vi "Measurement Logic.vi"(8 "error in":errorcluster, 9 "measurement configuration":T2 {"PAYLOAD" format="%x"; "TYPE" items=["CAN Data"=0, "CAN Remote"=1, "CAN Bus Error"=2, "CAN 2.0 Data"=8, "CAN FD Data"=16, "CAN FD+BRS Data"=24, "J1939 Data"=192, "Delay"=224, "Log Trigger"=225, "Start Trigger"=226]; "IDENTIFIER" format="%x"; "Baudrate" format="%x"; "FD Baudrate" format="%x"}, 10 "measure call context in":refnum<class "Measure Call Context.lvclass">) -> (0 "error out":errorcluster, 1 "measurement results":T1, 2 "measure call context out":refnum<class "Measure Call Context.lvclass">)   [LabVIEW 2025, in "CAN-LIN Frame Generator.lvclass"]
doc: "Contains the core logic for executing the measurement."
uses:
  CAN-LIN Frame Generator.lvclass
  <vilib>/Plug-In SDKs/Measurements/Measure Call Context/Measure Call Context.lvclass
  Measurement Configuration.ctl
  Measurement Results.ctl
  <vilib>/xnet/xnet.llb/XNET Frame CAN.ctl
  <vilib>/xnet/xnet.llb/XNET Frame Type CAN.ctl
  <vilib>/xnet/xnet.llb/XNET Create Session (Frame Output Stream).vi
  <vilib>/xnet/xnet.llb/XNET Write (Frame CAN).vi
  <vilib>/xnet/xnet.llb/XNET Wait (Transmit Complete).vi
  <extravilib>/ChannelInstances/Event Messenger-bool/Instantiate.vi
  <resource>/objmgr/xnet.rc
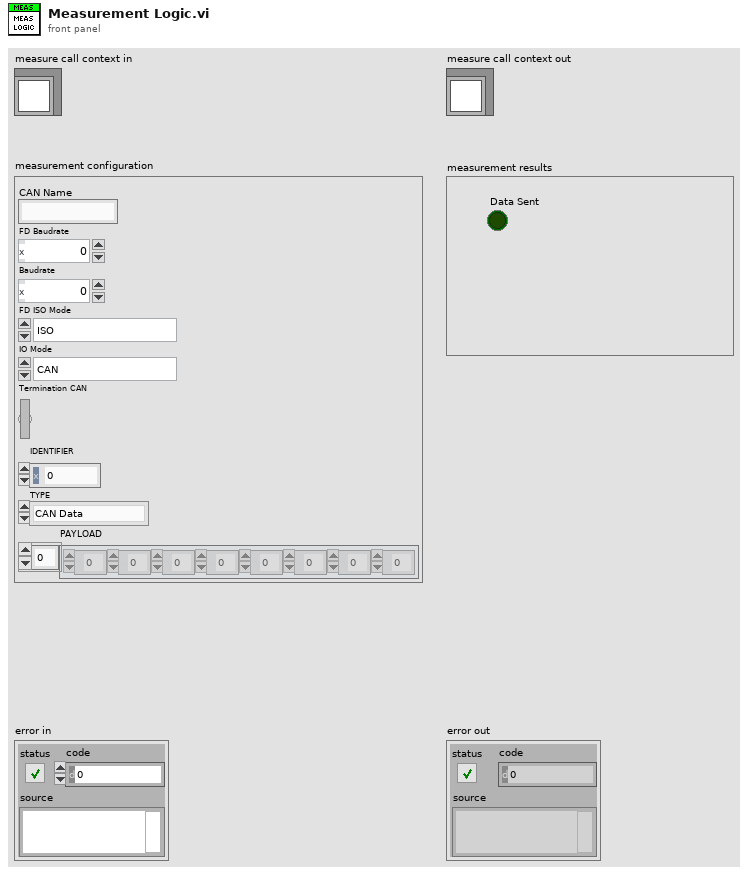
[diagram p1: front panel]
types:
  T1 = typedef "CAN-LIN Frame Generator.lvclass/Measurement Results.ctl" = cluster{"Data Sent":bool}
  T2 = typedef "CAN-LIN Frame Generator.lvclass/Measurement Configuration.ctl" = cluster{"CAN Name ":string, "FD Baudrate":u32, "Baudrate":u32, "FD ISO Mode":enum32{"ISO", "Legacy ISO", "Non-ISO"}, "IO Mode":enum32{"CAN", "CAN FD", "CAN FD + BRS"}, "Termination CAN":bool, "IDENTIFIER":u32, "TYPE":u32, "PAYLOAD":u32[]}
  T3 = typedef "XNET Frame CAN.ctl" = cluster{"timestamp":timestamp, "payload":u8[], "identifier":u32, "type":T4, "extended?":bool, "echo?":bool}
  T4 = typedef "XNET Frame Type CAN.ctl" = u8
  T5 = typedef "Event Messenger-bool.lvlib/))Channel.ctl" = refnum<queue>
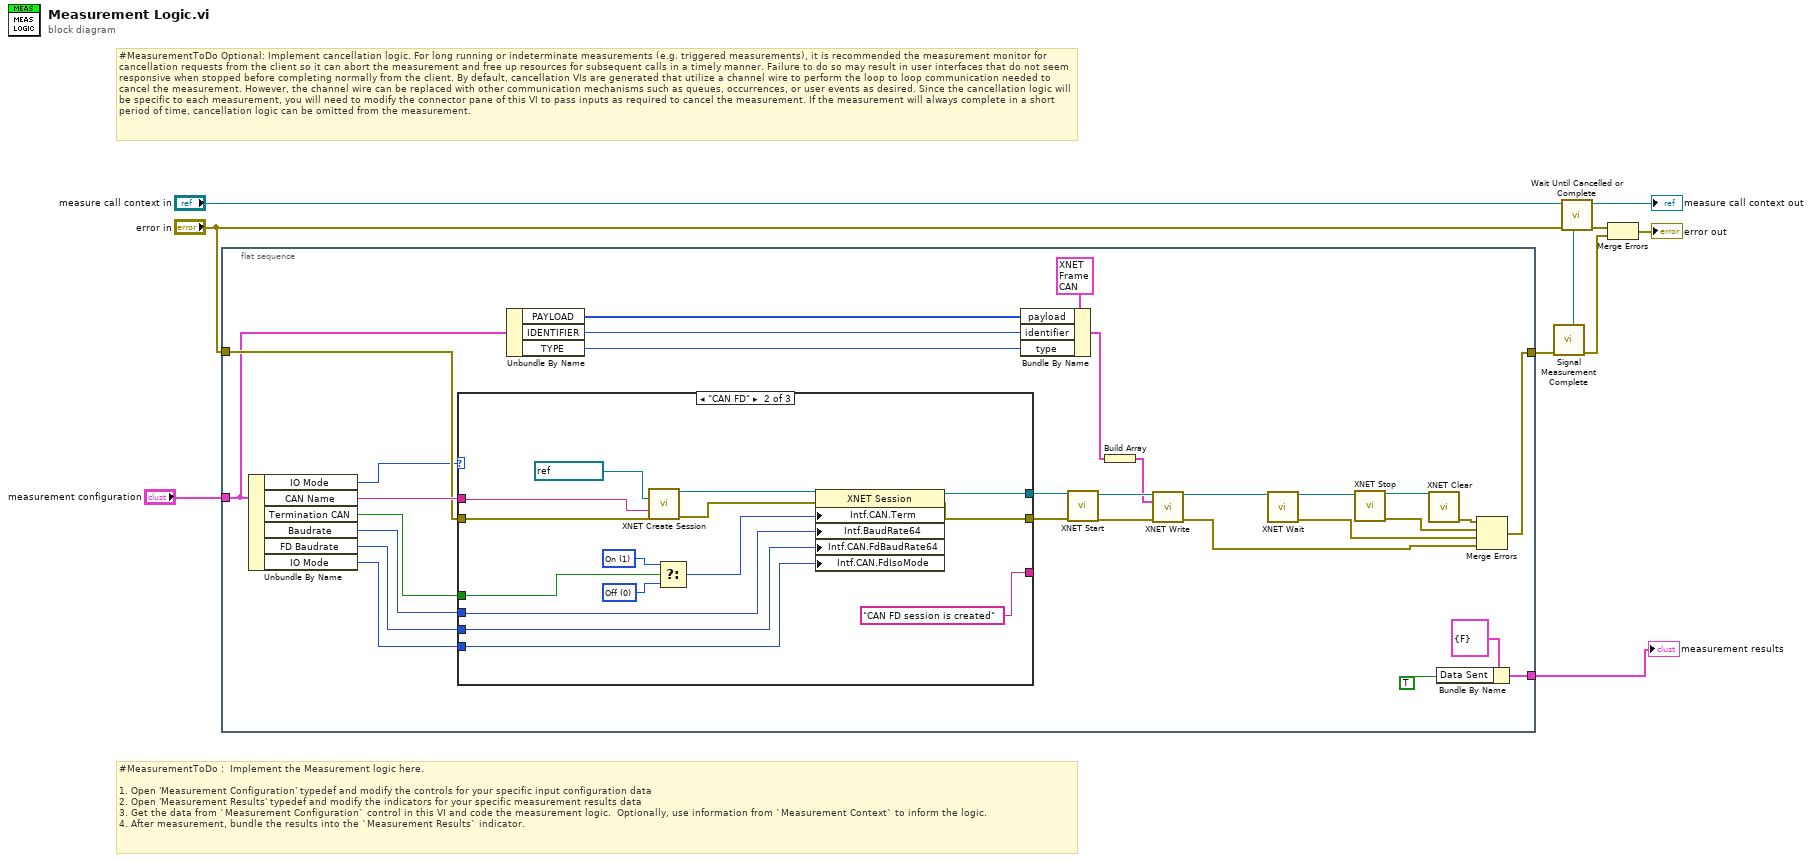
[diagram p0: block diagram]
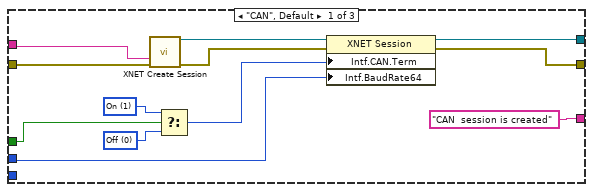
[diagram p2: hidden frame]
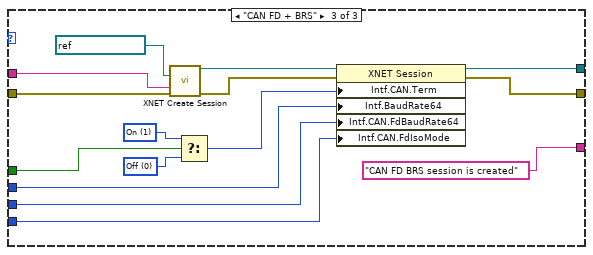
[diagram p3: hidden frame]
diagram:
  # "#MeasurementToDo Optional: Implement cancellation logic. For long running or indeterminate measurements (e.g. triggered measurements), it is recommended the measurement monitor for cancellation requests from the client so it can abort the measurement and free up resources for subsequent calls in a timely manner. Failure to do so may result in user interfaces that do not seem responsive when stopped before completing normally from the client. By default, cancellation VIs are generated that utilize a channel wire to perform the loop to loop communication needed to cancel the measurement. However, the channel wire can be replaced with other communication mechanisms such as queues, occurrences, or user events as desired. Since the cancellation logic will be specific to each measurement, you will need to modify the connector pane of this VI to pass inputs as required to cancel the measurement. If the measurement will always complete in a short period of time, cancellation logic can be omitted from the measurement."
  # "#MeasurementToDo :  Implement the Measurement logic here.\n\n1. Open 'Measurement Configuration' typedef and modify the controls for your specific input configuration data\n2. Open 'Measurement Results' typedef and modify the indicators for your specific measurement results data\n3. Get the data from `Measurement Configuration` control in this VI and code the measurement logic.  Optionally, use information from `Measurement Context` to inform the logic.\n4. After measurement, bundle the results into the `Measurement Results` indicator."
  n1 = flat-sequence {
    tunnel: "measurement configuration" -> [w14]
    tunnel: "error in" -> [w38]
    tunnel: [w16] -> w6
    tunnel: [w28] -> w1
    frame #0 {
      n2 = Unbundle By Name(w14) -> ("IO Mode"=w26:enum32{"CAN", "CAN FD", "CAN FD + BRS"}, "CAN Name"=w39:string, "Termination CAN"=w37:bool, "Baudrate"=w36:u32, "FD Baudrate"=w35:u32, "IO Mode"=w34:enum32{"CAN", "CAN FD", "CAN FD + BRS"})
      n3 = case shown="\"CAN FD\"" w26 {
        tunnel: [w46 w55 w75] -> w33
        tunnel: w39 -> [w41 w60 w70]
        tunnel: w38 -> [w45 w59 w69]
        tunnel: [w44 w54 w68] -> w32
        tunnel: w37 -> [w43 w58 w74]
        tunnel: w36 -> [w42 w57 w73]
        tunnel: w35 -> [_ w53 w72]
        tunnel: w34 -> [_ w56 w71]
        tunnel: ["CAN  session is created" ("message") "CAN FD session is created" ("message") "CAN FD BRS session is created" ("message")] -> _
        frame "CAN", Default {
          w49 = u32 1 items=["Off", "On"] ("Interface:CAN:Termination")
          w48 = u32 0 items=["Off", "On"] ("Interface:CAN:Termination")
          n4 = call-poly <vilib>:"XNET Create Session.vi"("interface"=w41, "error in (no error)"=w45) -> ("session out"=w51:refnum<k21>, "error out"=w50:errorcluster)  [unwired: 12 in]
          n5 = Select(t=w49, s=w43, f=w48) -> (s? t:f=w47:u32)
          n6 = property class="XNET Session"(reference=w51, error in=w50, "Intf.CAN.Term"=w47, "Intf.BaudRate64"=w42) -> (reference out=w46:refnum<k21>, error out=w44:errorcluster)
        }
        frame "CAN FD" {
          w63 = u32 1 items=["Off", "On"] ("Interface:CAN:Termination")
          w62 = u32 0 items=["Off", "On"] ("Interface:CAN:Termination")
          n7 = call-poly <vilib>:"XNET Create Session.vi"("cluster (:memory:)"=refnum<k21> ":can_fd:", "interface"=w60, "error in (no error)"=w59) -> ("session out"=w65:refnum<k21>, "error out"=w64:errorcluster)  [unwired: 11 in]
          n8 = Select(t=w63, s=w58, f=w62) -> (s? t:f=w61:u32)
          n9 = property class="XNET Session"(reference=w65, error in=w64, "Intf.CAN.Term"=w61, "Intf.BaudRate64"=w57, "Intf.CAN.FdBaudRate64"=w53, "Intf.CAN.FdIsoMode"=w56) -> (reference out=w55:refnum<k21>, error out=w54:errorcluster)
        }
        frame "CAN FD + BRS" {
          w78 = u32 1 items=["Off", "On"] ("Interface:CAN:Termination")
          w77 = u32 0 items=["Off", "On"] ("Interface:CAN:Termination")
          n10 = call-poly <vilib>:"XNET Create Session.vi"("cluster (:memory:)"=refnum<k21> ":can_fd_brs:", "interface"=w70, "error in (no error)"=w69) -> ("session out"=w80:refnum<k21>, "error out"=w79:errorcluster)  [unwired: 11 in]
          n11 = Select(t=w78, s=w74, f=w77) -> (s? t:f=w76:u32)
          n12 = property class="XNET Session"(reference=w80, error in=w79, "Intf.CAN.Term"=w76, "Intf.BaudRate64"=w73, "Intf.CAN.FdBaudRate64"=w72, "Intf.CAN.FdIsoMode"=w71) -> (reference out=w75:refnum<k21>, error out=w68:errorcluster)
        }
      }
      n13 = Unbundle By Name(w14) -> ("PAYLOAD"=w13:u32[], "IDENTIFIER"=w12:u32, "TYPE"=w11:u32)
      n14 = Bundle By Name(cluster=T3 {"timestamp"=timestamp(0 s since 1904-01-01), "payload"=[1, 2, 3, 4, 5, 6, 7, 8], "identifier"=2, "type"=0, "extended?"=FALSE, "echo?"=FALSE} ("CAN frame"), "payload"=w13, "identifier"=w12, "type"=w11) -> (w24:T3)
      n15 = call <vilib>:"XNET Start.vi"("session in"=w33, "error in (no error)"=w32) -> ("session out"=w31:refnum<k21>, "error out"=w30:errorcluster)  [unwired: 12 in]
      n16 = Build Array(w24) -> (w23:T3[])
      n17 = call-poly <vilib>:"XNET Write.vi"("session in"=w31, "data"=w23, "error in (no error)"=w30) -> ("session out"=w22:refnum<k21>, "error out"=w15:errorcluster)  [unwired: 11 out]
      n18 = call-poly <vilib>:"XNET Wait.vi"("session in"=w22) -> ("session out"=w21:refnum<k21>, "error out"=w17:errorcluster)  [unwired: 13 in]
      n19 = call <vilib>:"XNET Stop.vi"("session in"=w21) -> ("session out"=w20:refnum<k21>, "error out"=w18:errorcluster)  [unwired: 13 in]
      n20 = call <vilib>:"XNET Clear.vi"("session in"=w20) -> ("error out"=w19:errorcluster)  [unwired: 14 in]
      n21 = Bundle By Name(cluster=T1 {"Data Sent"=FALSE} ("measurement results"), "Data Sent"=TRUE) -> (w28:T1)
      n22 = Merge Errors(w19, w18, w17, w15) -> (w16:errorcluster)
    }
  }
  n23 = call "Signal Measurement Complete.vi"("error in (no error)"=w6) -> ("error out"=w4:errorcluster, "done channel"=w5:T5)  [unwired: 9 in]
  n24 = call "Wait Until Cancelled or Complete.vi"("done channel"=w5, "error in (no error)"="error in", "measure call context in"="measure call context in") -> ("error out"=w3:errorcluster, "measure call context out"=→"measure call context out":refnum<class "Measure Call Context.lvclass">)  [unwired: 7 in]
  n25 = Merge Errors(w3, w4) -> (→"error out":errorcluster)
  "measurement results" <- w1
